vi "Parse Content References.vi"(0 "file path in":path) -> (6 "transposed array":string[][](array[string]))   [LabVIEW 2026]
uses:
  <vilib>/LAVA/Robust CSV/Robust CSV.lvlib
panel:
  out "error IO":errorcluster
  in  "error in (no error)":errorcluster
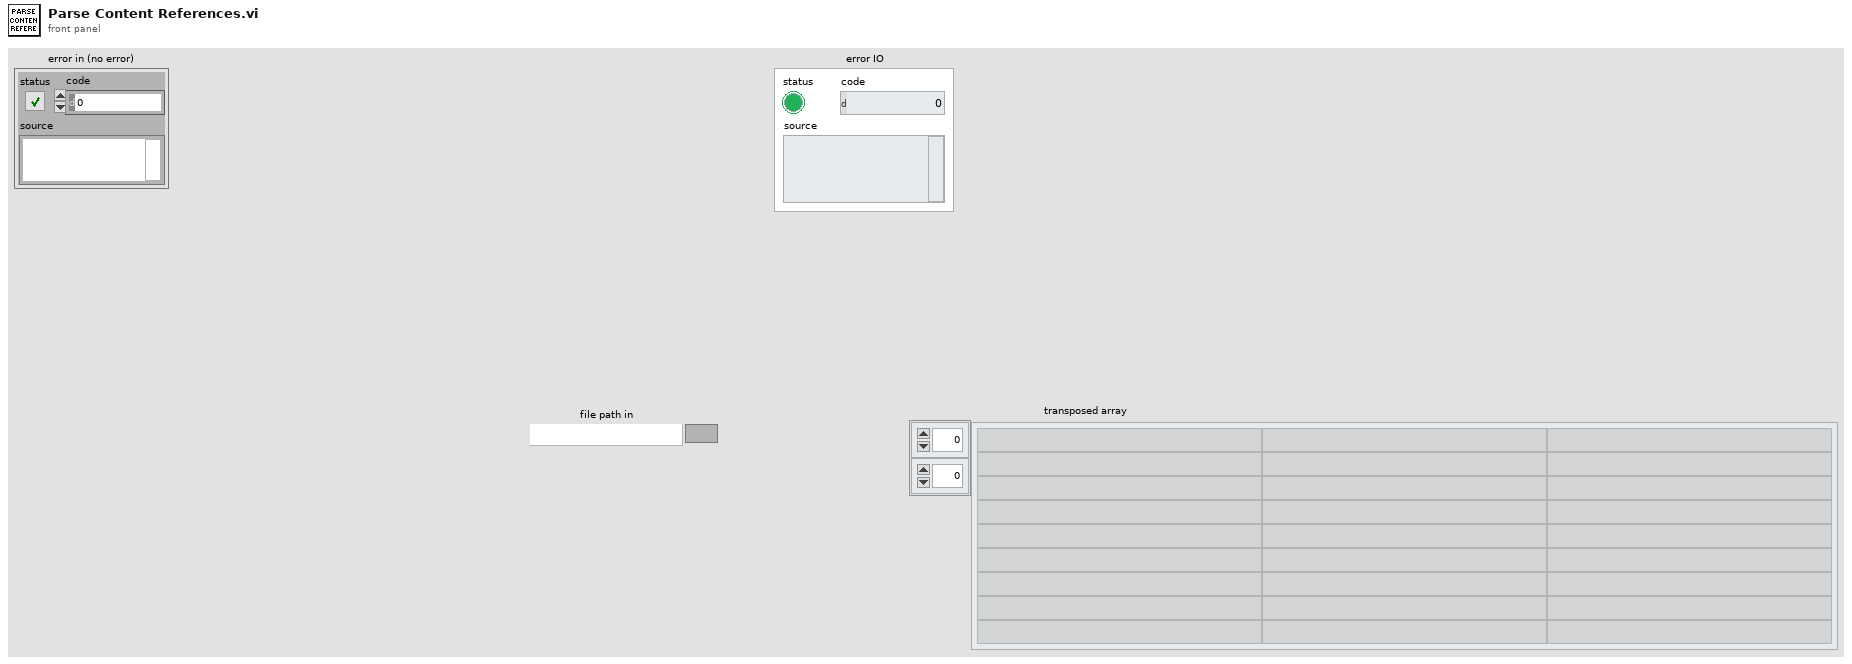
[diagram p1: front panel]
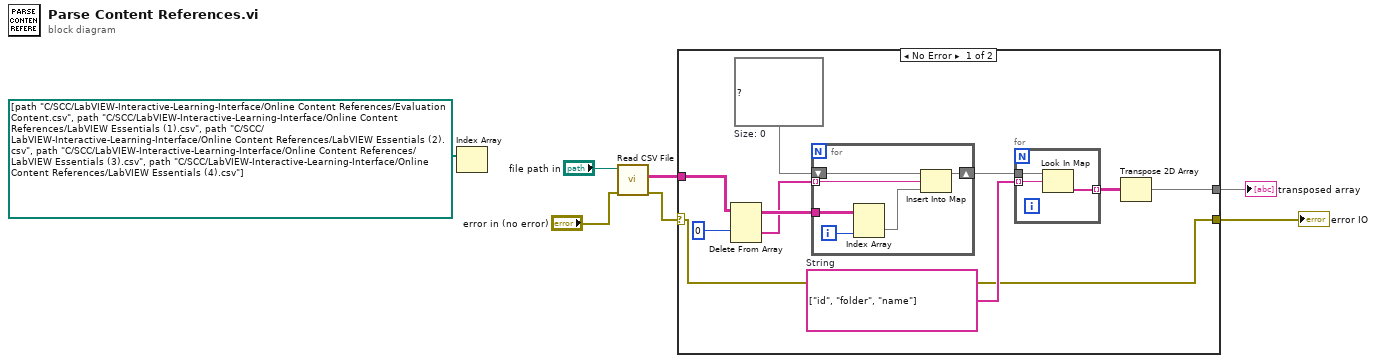
[diagram p0: block diagram]
diagram:
  n1 = Index Array(array=path[] [path "C:/SCC/LabVIEW-Interactive-Learning-Interface/Online Content References/Evaluation Content.csv", path "C:/SCC/LabVIEW-Interactive-Learning-Interface/Online Content References/LabVIEW Essentials (1).csv", path "C:/SCC/LabVIEW-Interactive-Learning-Interface/Online Content References/LabVIEW Essentials (2).csv", path "C:/SCC/LabVIEW-Interactive-Learning-Interface/Online Content References/LabVIEW Essentials (3).csv", path "C:/SCC/LabVIEW-Interactive-Learning-Interface/Online Content References/LabVIEW Essentials (4).csv"]) -> ()  [unwired: 1 in, 1 out]
  n2 = call <vilib>:"Read CSV File.vi"("error in (no error)"="error in (no error)", "file path in"="file path in") -> ("error out"=w2:errorcluster, "2-D array"=w5:string[][])  [unwired: 7 in, 1 out]
  n3 = case shown="No Error" w2 {
    selector: w2 -> [w8 w28]
    tunnel: [w10 w27] -> w6
    tunnel: w5 -> [w9 w27]
    tunnel: [w8 w28] -> w1
    frame No Error {
      w12 = string[] ["id", "folder", "name"]  # String
      w14 = map{string, string[]} {}  # Size: 0
      n4 = Delete From Array(array=w9, index (row)=0 ("index (col)")) -> (deleted portion=w15:string[], array with subset deleted=w17:string[][])  [unwired: 2 in]
      n5 = for {
        tunnel: w17 -> [w25]
        tunnel: w15 -> [w26] mode=indexing
        shift-right: [w22] -> w13
        shift-left: w14 -> [w21]
        i -> [w24]
        n6 = Index Array(array=w25, index (col)=w24) -> (element=w23:string[])  [unwired: 1 in]
        n7 = Insert Into Map(map in=w21, key=w26, value=w23) -> (map out=w22:map{string, string[]})  [unwired: 2 out]
      }
      n8 = for {
        tunnel: w13 -> [w20]
        tunnel: w12 -> [w19] mode=indexing
        tunnel: [w18] -> w11 mode=indexing
        n9 = Look In Map(map=w20, key=w19) -> (value=w18:string[])  [unwired: 1 in, 1 out]
      }
      n10 = Transpose 2D Array(2D array=w11) -> (transposed array=w10:string[][])
    }
    frame Error {
    }
  }
  "transposed array" <- w6
  "error IO" <- w1
